vi "test_add_elements.vi"() -> ()   [LabVIEW 2016]
uses:
  add_element(array).vi
  add_element(variant).vi
panel:
  out "elapsed time in millisec (variant)":dbl
  out "elapsed time in millisec (array)":dbl
  in  "number of elements":i32=10000
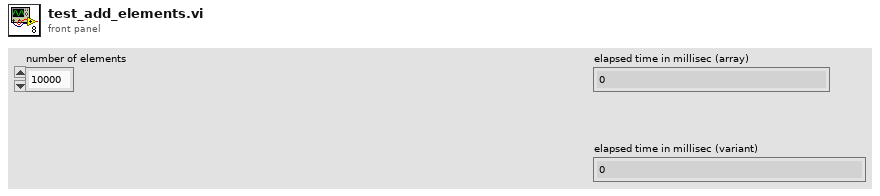
[diagram p1: front panel]
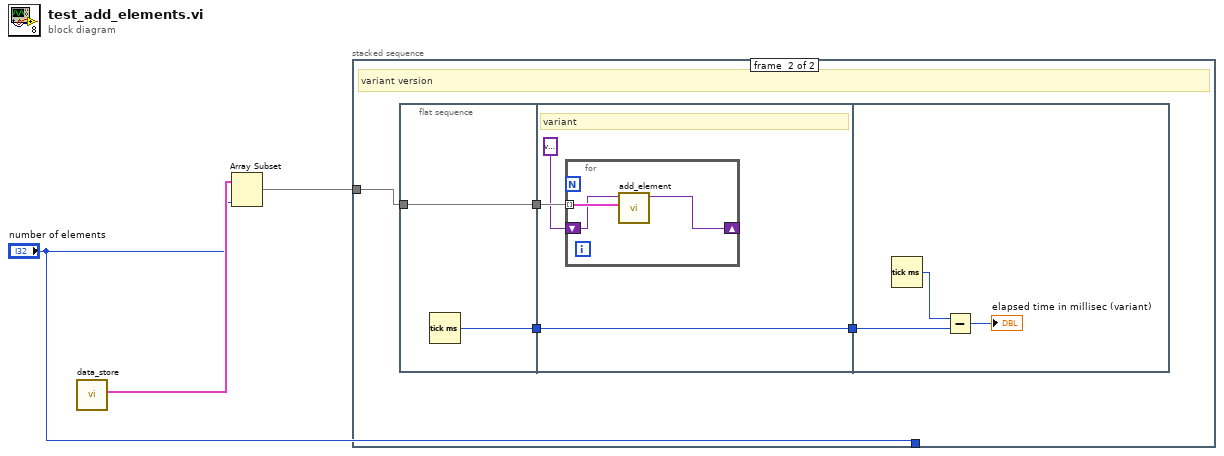
[diagram p0: block diagram]
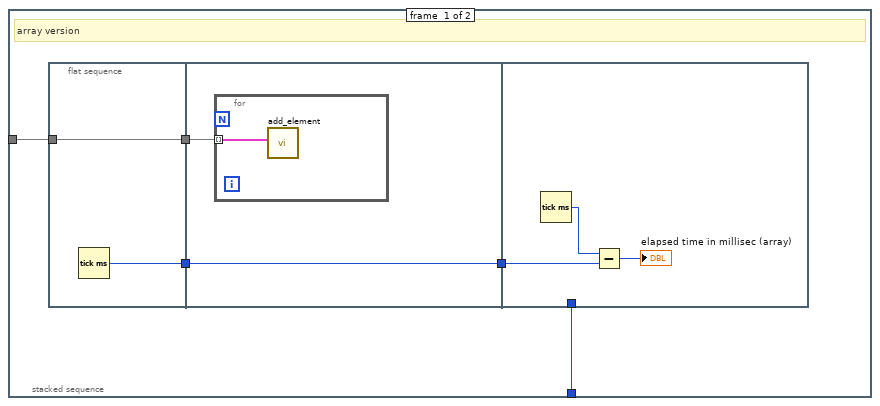
[diagram p2: hidden frame]
diagram:
  n1 = call "data_store.vi"() -> ("array items"=w3:cluster{"name":string, "address":string}[])  [unwired: 10 in, 1 out]
  n2 = Array Subset(array=w3, length="number of elements") -> (w1:cluster{"name":string, "address":string}[])  [unwired: 1 in]
  n3 = stacked-sequence {
    tunnel: "number of elements" -> [w5 _]
    tunnel: w1 -> [w4 w17]
    frame #0 {
      # "array version"
      n4 = flat-sequence {
        tunnel: [w10] -> w8
        tunnel: w4 -> [w9]
        tunnel: [w9] -> w7
        tunnel: [w12] -> w6
        tunnel: w8 -> [w12]
        tunnel: w7 -> [w11]
        tunnel: w6 -> [w15]
        tunnel: w5 -> [_]
        frame #0 {
          n5 = Tick Count (ms)() -> (millisecond timer value=w10:u32)
        }
        frame #1 {
          n6 = for {
            tunnel: w11 -> [w13] mode=indexing
            n7 = call-poly "add_element.vi"("element"=w13) -> ()  [unwired: 9 in, 2 out]
          }
        }
        frame #2 {
          n8 = Tick Count (ms)() -> (millisecond timer value=w16:u32)
          n9 = Subtract(x=w16, y=w15) -> (x-y=→"elapsed time in millisec (array)":u32)
        }
      }
    }
    frame #1 {
      # "variant version"
      n10 = flat-sequence {
        tunnel: [w22] -> w20
        tunnel: w17 -> [w21]
        tunnel: [w21] -> w19
        tunnel: [w25] -> w18
        tunnel: w20 -> [w25]
        tunnel: w19 -> [w24]
        tunnel: w18 -> [w30]
        frame #0 {
          n11 = Tick Count (ms)() -> (millisecond timer value=w22:u32)
        }
        frame #1 {
          # "variant"
          n12 = for {
            tunnel: w24 -> [w28] mode=indexing
            shift-right: [w26] -> _
            shift-left: variant ("data store (variant)") -> [w27]
            n13 = call-poly "add_element.vi"("element"=w28, "data store (variant)"=w27) -> ("data store (variant)"=w26:variant)  [unwired: 8 in, 1 out]
          }
        }
        frame #2 {
          n14 = Tick Count (ms)() -> (millisecond timer value=w31:u32)
          n15 = Subtract(x=w31, y=w30) -> (x-y=→"elapsed time in millisec (variant)":u32)
        }
      }
    }
  }
